vi "Get User Interface VI.vi"(8 "error in (no error)":errorcluster, 11 "RDMA Plugin User Interface in":refnum<class "RDMA Plugin User Interface.lvclass">) -> (0 "error out":errorcluster, 2 "user interface vi":refnum<vi>, 3 "RDMA Plugin User Interface out":refnum<class "RDMA Plugin User Interface.lvclass">)   [LabVIEW 2020, in "RDMA.lvlib" / "RDMA Plugin User Interface.lvclass"]
uses:
  RDMA Plugin User Interface.lvclass
  User Interface.vi
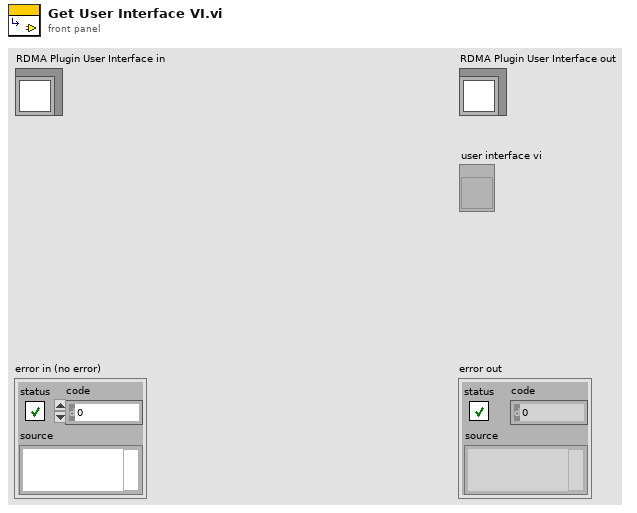
[diagram p1: front panel]
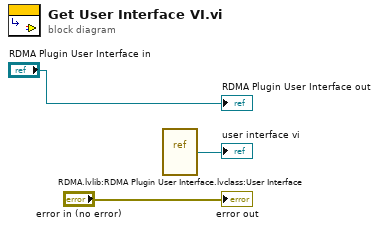
[diagram p0: block diagram]
diagram:
  n1 = vi-ref "RDMA.lvlib:RDMA Plugin User Interface.lvclass:User Interface.vi"() -> (→"user interface vi":refnum<vi>)
  "error out" <- "error in (no error)"
  "RDMA Plugin User Interface out" <- "RDMA Plugin User Interface in"
